vi "Create SubAddress Name from Address.vi"(11 "Address":string) -> (3 "SA name out":string)   [LabVIEW 2020, in "Configuration_Helper.lvlib"]
uses:
  Configuration_Helper.lvlib
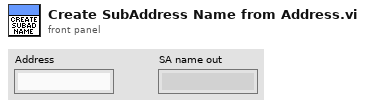
[diagram p1: front panel]
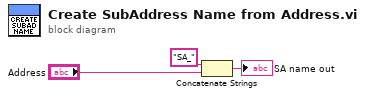
[diagram p0: block diagram]
diagram:
  n1 = Concatenate Strings("SA_" ("string"), "Address") -> (→"SA name out":string)
